vi "Router - Close.vi"(8 "error in (no error)":errorcluster, 11 "Router Data In":T1) -> (0 "error out":errorcluster)   [LabVIEW 2016, in "PXImc Router.lvlib"]
uses:
  PXImc Router.lvlib
  Controls/Router - Configuration.ctl
  Controls/Router/Node Block R-W Properties.ctl
  Controls/Router/Block Properties.ctl
  Controls/Router/Router - PXImc Properties.ctl
  Controls/Router/Router - PXImc Card Properties.ctl
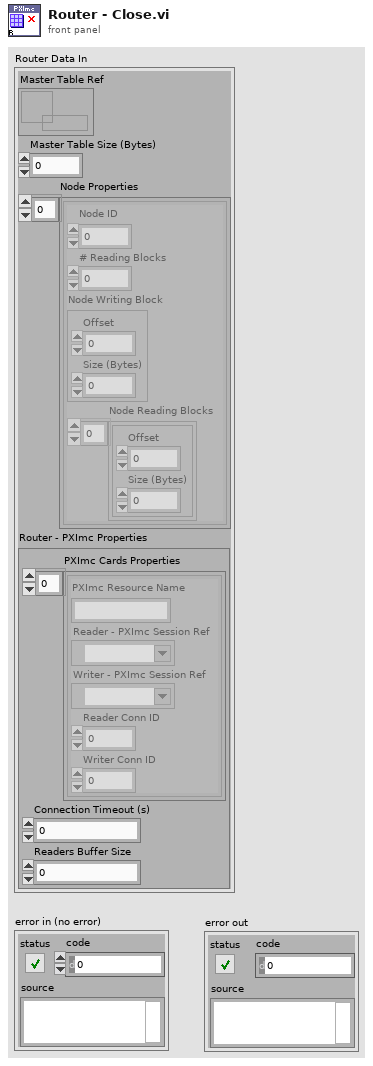
[diagram p1: front panel]
types:
  T1 = typedef "PXImc Router.lvlib/Router - Configuration.ctl" = cluster{"Master Table Ref":refnum<data-value>, "Master Table Size (Bytes)":u32, "Node Properties":T2[], "Router - PXImc Properties":T4}
  T2 = typedef "PXImc Router.lvlib/Node Block R-W Properties.ctl" = cluster{"Node ID":u32, "# Reading Blocks":u32, "Node Writing Block":T3, "Node Reading Blocks":T3[]}
  T3 = typedef "PXImc Router.lvlib/Block Properties.ctl" = cluster{"Offset":u32, "Size (Bytes)":u32}
  T4 = typedef "PXImc Router.lvlib/Router - PXImc Properties.ctl" = cluster{"PXImc Cards Properties":T5[], "Connection Timeout (s)":dbl, "Readers Buffer Size":u64}
  T5 = typedef "PXImc Router.lvlib/Router - PXImc Card Properties.ctl" = cluster{"PXImc Resource Name":string, "Reader - PXImc Session Ref":refnum<k21>, "Writer - PXImc Session Ref":refnum<k21>, "Reader Conn ID":u16, "Writer Conn ID":u16}
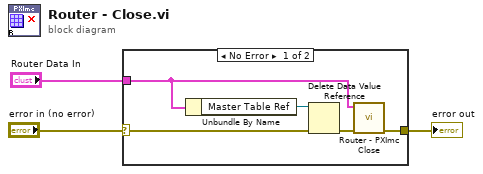
[diagram p0: block diagram]
diagram:
  n1 = case shown="No Error" "error in (no error)" {
    selector: "error in (no error)" -> [w7 w9]
    tunnel: [w4 w9] -> w3
    tunnel: "Router Data In" -> [w6 _]
    frame No Error {
      n2 = Unbundle By Name(w6) -> ("Master Table Ref"=w8:refnum<data-value>)
      n3 = Delete Data Value Reference(data value reference=w8, error in=w7) -> (error out=w5:errorcluster)  [unwired: 1 out]
      n4 = call "Router - PXImc Close.vi"("error in (no error)"=w5, "Router Data In"=w6) -> ("error out"=w4:errorcluster)  [unwired: 9 in]
    }
    frame Error {
    }
  }
  "error out" <- w3
